vi "GT_SetCaptureSense.vi"(3 "sense":i16, 4 "Mode":u16(ring) items=["Home", "Index", "Probe"], 5 "encode":i16, 6 "rtn_In":cluster{"rtn":i16, "Func":string}) -> (1 "encode out":i16, 2 "rtn_Out":cluster{"rtn":i16, "Func":string})   [LabVIEW 2014]
uses:
  VC6/gts.dll
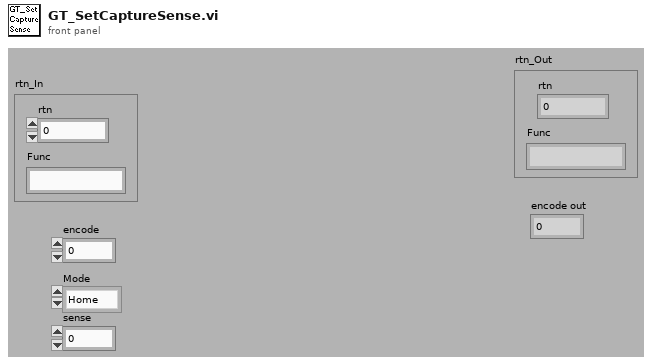
[diagram p1: front panel]
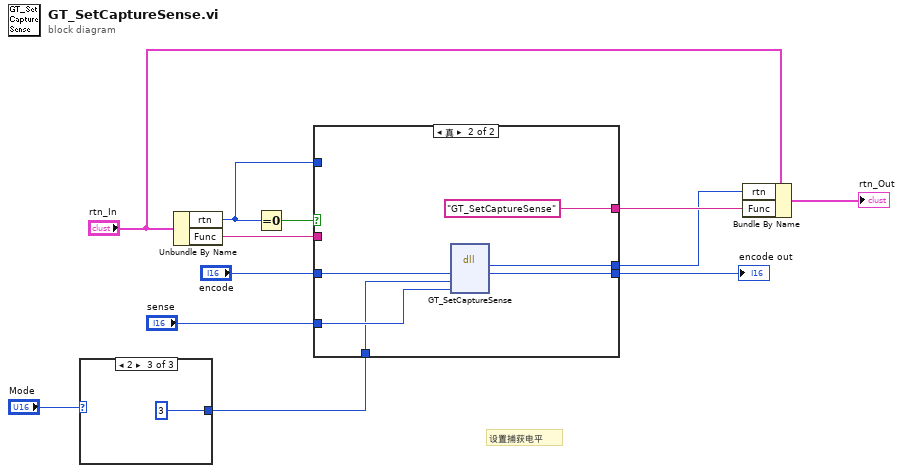
[diagram p0: block diagram]
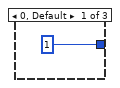
[diagram p2: hidden frame]
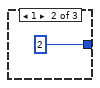
[diagram p3: hidden frame]
diagram:
  # "设置捕获电平"
  n1 = case shown="2" "Mode" {
    tunnel: [i16 1 ("mode") i16 2 ("mode") i16 3 ("mode")] -> w2
    frame 0, Default {
    }
    frame 1 {
    }
    frame 2 {
    }
  }
  n2 = Unbundle By Name("rtn_In") -> ("rtn"=w7:i16, "Func"=w6:string)
  n3 = Equal To 0?(x=w7) -> (x = 0?=w12:bool)
  n4 = case shown="真" w12 {
    tunnel: [w17 "GT_SetCaptureSense" ("Func")] -> w9
    tunnel: [w18 w23] -> w8
    tunnel: w7 -> [w18 _]
    tunnel: w6 -> [w17 _]
    tunnel: "encode" -> [w16 w22]
    tunnel: "sense" -> [_ w21]
    tunnel: w2 -> [_ w20]
    tunnel: [w16 w19] -> w1
    frame False {
    }
    frame True {
      n5 = dll-call lib="PTH2Fabs DNewGTS AC-800LWin7版源程序-20170926gts85VC6gts.dll" fn="GT_SetCaptureSense"("encode"=w22, "mode"=w20, "sense"=w21) -> ("rtn"=w23:i16, "encode"=w19:i16)  [unwired: 5 in, 2 out]
    }
  }
  "encode out" <- w1
  n6 = Bundle By Name(cluster="rtn_In", "rtn"=w8, "Func"=w9) -> (→"rtn_Out":cluster{"rtn":i16, "Func":string})
